vi "sync_write.vi"() -> ()   [LabVIEW 2016]
uses:
  dxl_x86_c.lvlib/dxl_x86_c.lvlib
panel:
  out "dynamixel_error":string
  out "dynamixel_comm_result":string
  out "group_num":i32
  in  "LEN_MX_\nGOAL_POSITION":u16=2
  out "value : MX (knob)\npresent position 2":u16(knob)
  in  "dynamixe2_id":u8=2
  in  "device_name":string="COM1"
  in  "ADDR_MX_\nPRESENT_POSITION":u16=36
  in  "ADDR_MX_\nGOAL_POSITION":u16=30
  in  "ADDR_MX_\nTORQUE_ENABLE":u16=24
  out "protocol_version":dbl=1.0
  out "value : MX (knob)\npresent position 1":u16(knob)
  in  "terminate":bool
  out "port_num":i32
  in  "value : MX (dial)\ngoal position":u16(knob)
  in  "dynamixel1_id":u8=1
  in  "baud_rate":i32=57600
  # "/*******************************************************************************\n* Copyright (c) 2016, ROBOTIS CO., LTD.\n* All rights reserved.\n*\n* Redistribution and use in source and binary forms, with or without\n* modification, are permitted provided that the following conditions are met:\n*\n* * Redistributions of source code must retain the above copyright notice, this\n*   list of conditions and the following disclaimer.\n*\n* * Redistributions in binary form must reproduce the above copyright notice,\n*   this list of conditions and the following disclaimer in the documentation\n*   and/or other materials provided with the distribution.\n*\n* * Neither the name of ROBOTIS nor the names of its\n*   contributors may be used to endorse or promote products derived from\n*   this software without specific prior written permission.\n*\n* THIS SOFTWARE IS PROVIDED BY THE COPYRIGHT HOLDERS AND CONTRIBUTORS \"AS IS\"\n* AND ANY EXPRESS OR IMPLIED WARRANTIES, INCLUDING, BUT NOT LIMITED TO, THE\n* IMPLIED WARRANTIES OF MERCHANTABILITY AND FITNESS FOR A PARTICULAR PURPOSE ARE\n* DISCLAIMED. IN NO EVENT SHALL THE COPYRIGHT HOLDER OR CONTRIBUTORS BE LIABLE\n* FOR ANY DIRECT, INDIRECT, INCIDENTAL, SPECIAL, EXEMPLARY, OR CONSEQUENTIAL\n* DAMAGES (INCLUDING, BUT NOT LIMITED TO, PROCUREMENT OF SUBSTITUTE GOODS OR\n* SERVICES; LOSS OF USE, DATA, OR PROFITS; OR BUSINESS INTERRUPTION) HOWEVER\n* CAUSED AND ON ANY THEORY OF LIABILITY, WHETHER IN CONTRACT, STRICT LIABILITY,\n* OR TORT (INCLUDING NEGLIGENCE OR OTHERWISE) ARISING IN ANY WAY OUT OF THE USE\n* OF THIS SOFTWARE, EVEN IF ADVISED OF THE POSSIBILITY OF SUCH DAMAGE.\n*******************************************************************************/\n\n/* Author: Ryu Woon Jung (Leon) */"
  # "Available Dynamixel model on this example : All models using Protocol 1.0\nThis example is designed for using two Dynamixel MX-28s, and an USB2DYNAMIXEL.\nTo use another Dynamixel model, such as X series, see their details in E-Manual(support.robotis.com) \n   and edit \"numeric control\"s seen left with \"Edit Text\" tool.\nBe sure that Dynamixel MX properties are already set as %% ID : 1 / Baudnum : 34 (Baudrate : 57600)\n\n1. Run example by click above \"Run\" button (below \"Edit\" menu).\n2. Drag \"dial\" then you may see the Dynamixel and \"knob\"s rotating\n3. To finish the example, press \"terminate\" button."
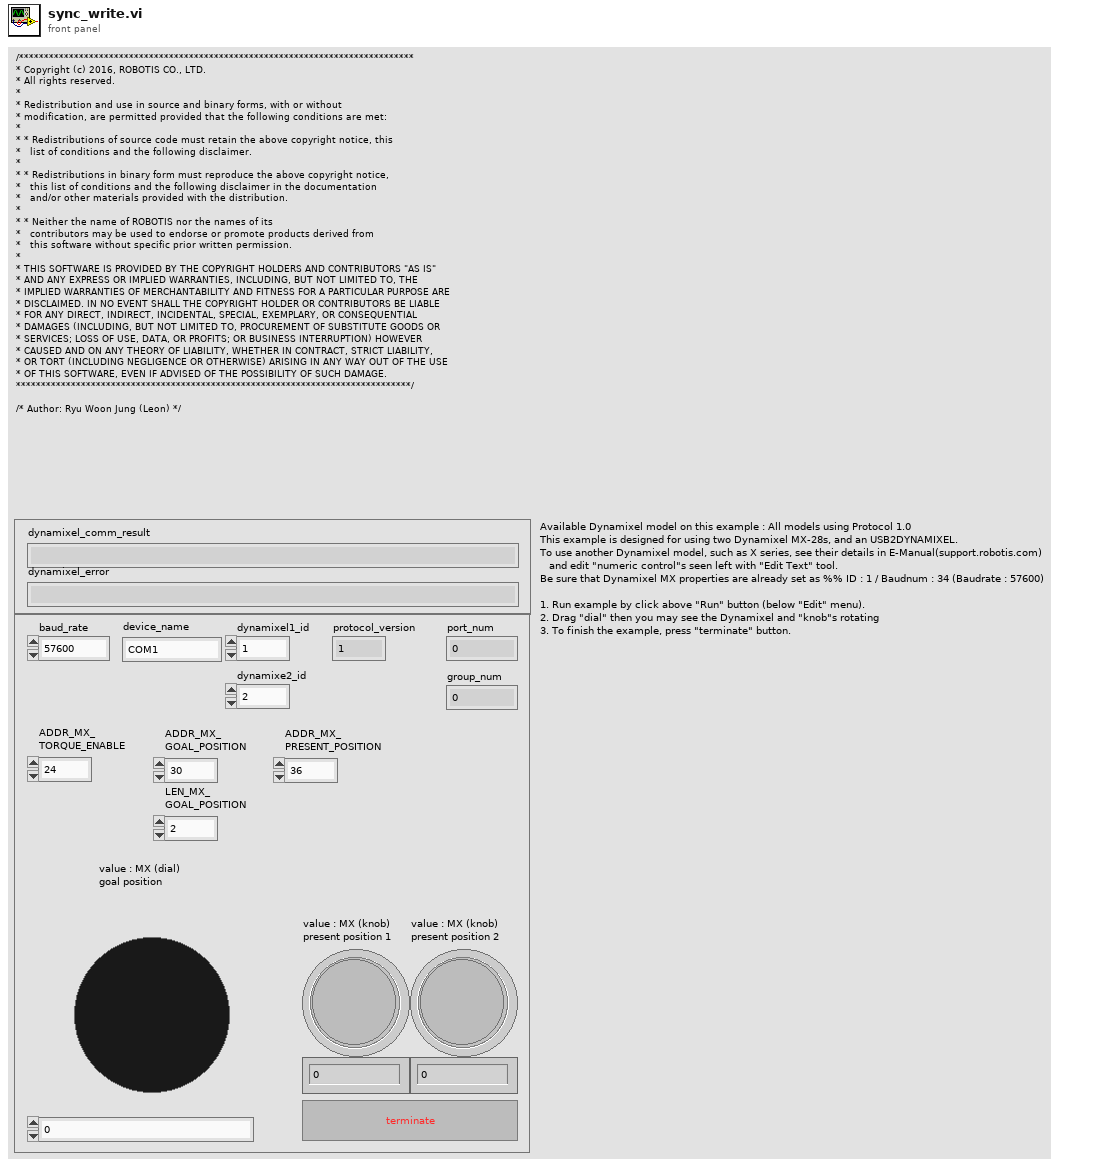
[diagram p1: front panel]
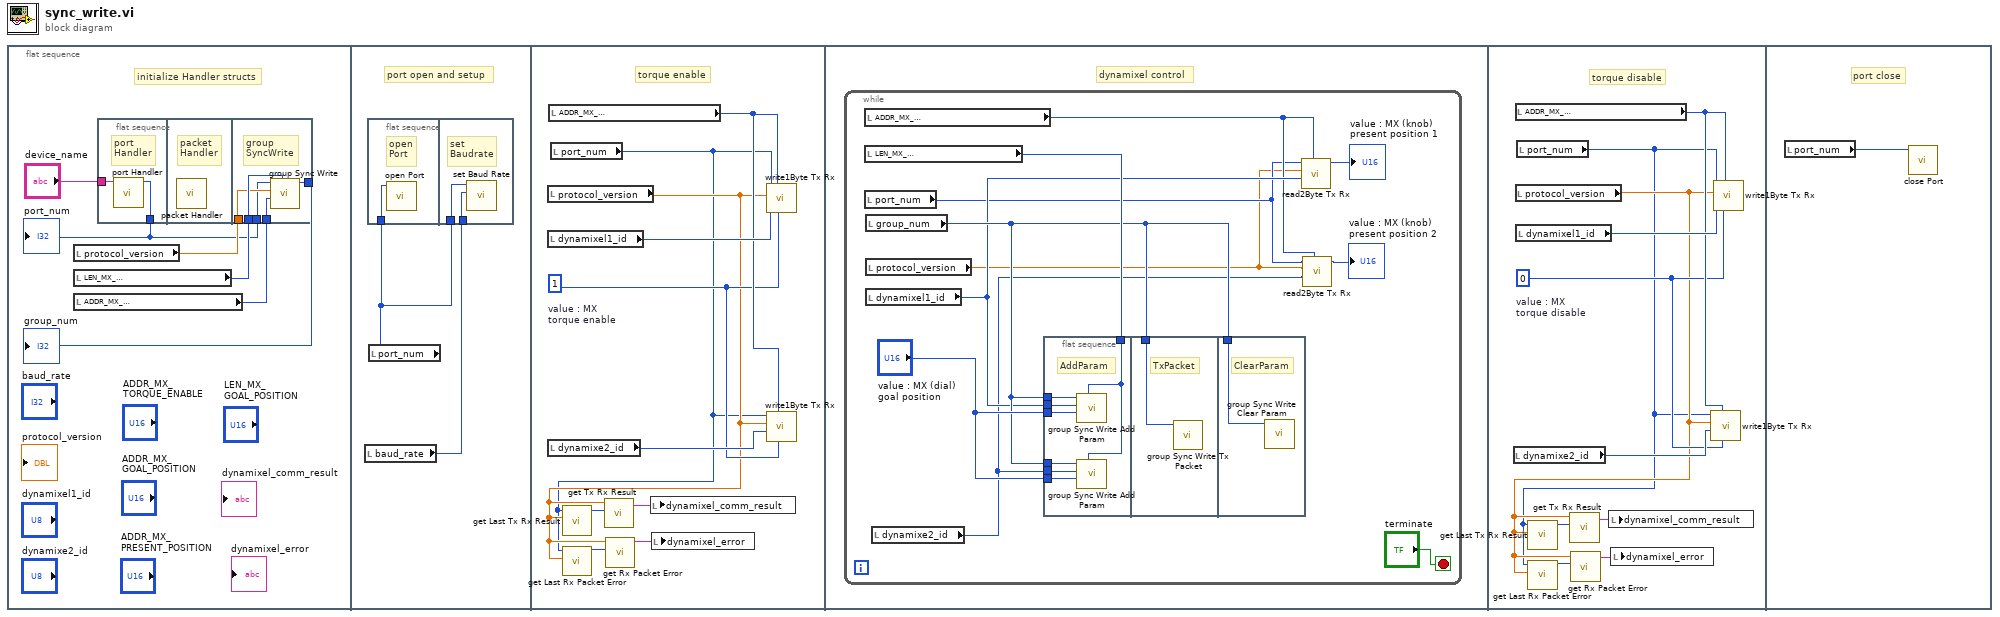
[diagram p0: block diagram]
diagram:
  n1 = flat-sequence {
    frame #0 {
      # "initialize Handler structs"
      n2 = local read "protocol_version"() -> (w3:dbl)
      n3 = local read "LEN_MX_\nGOAL_POSITION"() -> (w5:u16)
      n4 = local read "ADDR_MX_\nGOAL_POSITION"() -> (w4:u16)
      n5 = flat-sequence {
        tunnel: "device_name" -> [w8]
        tunnel: [w7] -> w2
        tunnel: w5 -> [w13]
        tunnel: w4 -> [w12]
        tunnel: w3 -> [w11]
        tunnel: w2 -> [w10]
        tunnel: [w9] -> w1
        frame #0 {
          # "port\nHandler"
          n6 = call "port Handler.vi"("port_name"=w8) -> ("function return"=w7:i32)  [unwired: 10 in]
        }
        frame #1 {
          # "packet\nHandler"
          n7 = call "packet Handler.vi"() -> ()  [unwired: 12 in]
        }
        frame #2 {
          # "group\nSyncWrite"
          n8 = call "group Sync Write.vi"("data_length"=w13, "start_address"=w12, "protocol_version"=w11, "port_num"=w10) -> ("function return"=w9:i32)  [unwired: 7 in]
        }
      }
      "port_num" <- w2
      "group_num" <- w1
    }
    frame #1 {
      # "port open and setup"
      n9 = local read "baud_rate"() -> (w14:i32)
      n10 = flat-sequence {
        tunnel: w15 -> [w16]
        tunnel: w15 -> [w18]
        tunnel: w14 -> [w17]
        frame #0 {
          # "open\nPort"
          n11 = call "open Port.vi"("port_num"=w16) -> ()  [unwired: 10 in, 1 out]
        }
        frame #1 {
          # "set\nBaudrate"
          n12 = call "set Baud Rate.vi"("baudrate"=w17, "port_num"=w18) -> ()  [unwired: 9 in, 1 out]
        }
      }
      n13 = local read "port_num"() -> (w15:i32)
    }
    frame #2 {
      w25 = 1  # value : MX torque enable
      # "torque enable"
      n14 = local read "protocol_version"() -> (w20:dbl)
      n15 = local read "dynamixel1_id"() -> (w28:u8)
      n16 = local read "dynamixe2_id"() -> (w26:u8)
      n17 = local read "ADDR_MX_\nTORQUE_ENABLE"() -> (w27:u16)
      n18 = local read "port_num"() -> (w19:i32)
      n19 = call "get Last Tx Rx Result.vi"("protocol_version"=w20, "port_num"=w19) -> ("function return"=w21:i32)  [unwired: 9 in]
      n20 = call "get Last Rx Packet Error.vi"("protocol_version"=w20, "port_num"=w19) -> ("function return"=w22:u8)  [unwired: 9 in]
      n21 = call "get Tx Rx Result.vi"("result"=w21, "protocol_version"=w20) -> ("function return"=w24:string)  [unwired: 9 in]
      n22 = call "get Rx Packet Error.vi"("error"=w22, "protocol_version"=w20) -> ("function return"=w23:string)  [unwired: 9 in]
      n23 = local write "dynamixel_comm_result"(w24) -> ()
      n24 = local write "dynamixel_error"(w23) -> ()
      n25 = call "write1Byte Tx Rx.vi"("data"=w25, "address"=w27, "id"=w28, "protocol_version"=w20, "port_num"=w19) -> ()  [unwired: 7 in]
      n26 = call "write1Byte Tx Rx.vi"("data"=w25, "address"=w27, "id"=w26, "protocol_version"=w20, "port_num"=w19) -> ()  [unwired: 7 in]
    }
    frame #3 {
      # "dynamixel control"
      n27 = while {
        stop <- "terminate" stop-if-true
        n28 = local read "ADDR_MX_\nPRESENT_POSITION"() -> (w34:u16)
        n29 = local read "LEN_MX_\nGOAL_POSITION"() -> (w38:u16)
        n30 = local read "port_num"() -> (w33:i32)
        n31 = local read "group_num"() -> (w36:i32)
        n32 = local read "protocol_version"() -> (w32:dbl)
        n33 = local read "dynamixel1_id"() -> (w35:u8)
        n34 = local read "dynamixe2_id"() -> (w31:u8)
        n35 = flat-sequence {
          tunnel: w38 -> [w46]
          tunnel: w36 -> [w45]
          tunnel: w36 -> [w44]
          tunnel: w35 -> [w43]
          tunnel: w31 -> [w42]
          tunnel: "value : MX (dial)\ngoal position" -> [w41]
          tunnel: "value : MX (dial)\ngoal position" -> [w40]
          tunnel: w36 -> [w47]
          tunnel: w36 -> [w48]
          frame #0 {
            # "AddParam"
            n36 = call "group Sync Write Add Param.vi"("data_length"=w46, "data"=w40, "id"=w43, "group_num"=w45) -> ()  [unwired: 7 in, 1 out]
            n37 = call "group Sync Write Add Param.vi"("data_length"=w46, "data"=w41, "id"=w42, "group_num"=w44) -> ()  [unwired: 7 in, 1 out]
          }
          frame #1 {
            # "TxPacket"
            n38 = call "group Sync Write Tx Packet.vi"("group_num"=w47) -> ()  [unwired: 11 in]
          }
          frame #2 {
            # "ClearParam"
            n39 = call "group Sync Write Clear Param.vi"("group_num"=w48) -> ()  [unwired: 11 in]
          }
        }
        n40 = call "read2Byte Tx Rx.vi"("address"=w34, "id"=w35, "protocol_version"=w32, "port_num"=w33) -> ("function return"=→"value : MX (knob)\npresent position 1":u16)  [unwired: 7 in]
        n41 = call "read2Byte Tx Rx.vi"("address"=w34, "id"=w31, "protocol_version"=w32, "port_num"=w33) -> ("function return"=→"value : MX (knob)\npresent position 2":u16)  [unwired: 7 in]
      }
    }
    frame #4 {
      w55 = 0  # value : MX torque disable
      # "torque disable"
      n42 = local read "dynamixe2_id"() -> (w56:u8)
      n43 = local read "ADDR_MX_\nTORQUE_ENABLE"() -> (w57:u16)
      n44 = local read "protocol_version"() -> (w50:dbl)
      n45 = local read "dynamixel1_id"() -> (w58:u8)
      n46 = local read "port_num"() -> (w49:i32)
      n47 = call "get Last Tx Rx Result.vi"("protocol_version"=w50, "port_num"=w49) -> ("function return"=w52:i32)  [unwired: 9 in]
      n48 = call "get Last Rx Packet Error.vi"("protocol_version"=w50, "port_num"=w49) -> ("function return"=w51:u8)  [unwired: 9 in]
      n49 = call "get Tx Rx Result.vi"("result"=w52, "protocol_version"=w50) -> ("function return"=w53:string)  [unwired: 9 in]
      n50 = call "get Rx Packet Error.vi"("error"=w51, "protocol_version"=w50) -> ("function return"=w54:string)  [unwired: 9 in]
      n51 = local write "dynamixel_comm_result"(w53) -> ()
      n52 = local write "dynamixel_error"(w54) -> ()
      n53 = call "write1Byte Tx Rx.vi"("data"=w55, "address"=w57, "id"=w56, "protocol_version"=w50, "port_num"=w49) -> ()  [unwired: 7 in]
      n54 = call "write1Byte Tx Rx.vi"("data"=w55, "address"=w57, "id"=w58, "protocol_version"=w50, "port_num"=w49) -> ()  [unwired: 7 in]
    }
    frame #5 {
      # "port close"
      n55 = local read "port_num"() -> (w59:i32)
      n56 = call "close Port.vi"("port_num"=w59) -> ()  [unwired: 11 in]
    }
  }
